vi "Update Message[ ].vi"(8 "error in (no error)":errorcluster, 10 "Message":variant, 11 "Telegram Class in":refnum<class "Telegram Class.lvclass">) -> (0 "error out":errorcluster, 3 "Telegram Class out":refnum<class "Telegram Class.lvclass">)   [LabVIEW 2015, in "Telegram Library.lvlib" / "Telegram Class.lvclass"]
doc: "Created IvanLis by LabVIEW Portal\nProfile: http://labviewportal.org/memberlist.php?mode=viewprofile&u=987\neMail: IvanLisanov@gMail.com\nTelegram: https://t.me/IvanLis"
uses:
  Telegram Class.lvclass
  JSON Library/TypeDef/Message Text.ctl
  TypeDef/Message.ctl
  Telegram Class.lvclass/Telegram Class.ctl
  Telegram Library.lvlib
  JSON Library/JSON Library.lvlib
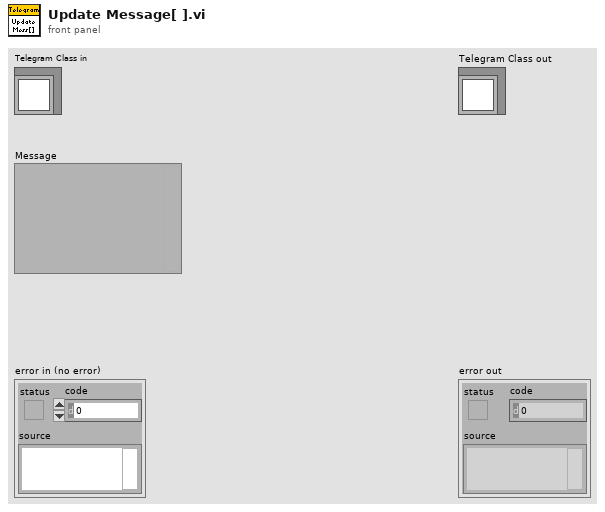
[diagram p1: front panel]
types:
  T1 = typedef "JSON Library.lvlib/Message Text.ctl" = cluster{"@type":string, "id":i64, "sender_id":cluster{"@type":string, "user_id":i64}, "chat_id":i64, "date":i64, "content":cluster{"@type":string, "text":cluster{"@type":string, "text":string}}}
  T2 = typedef "Telegram Library.lvlib/Message.ctl" = cluster{"id":i64, "chat_id":i64, "sender_user_id":i64, "date UTC":timestamp, "content_text":string}
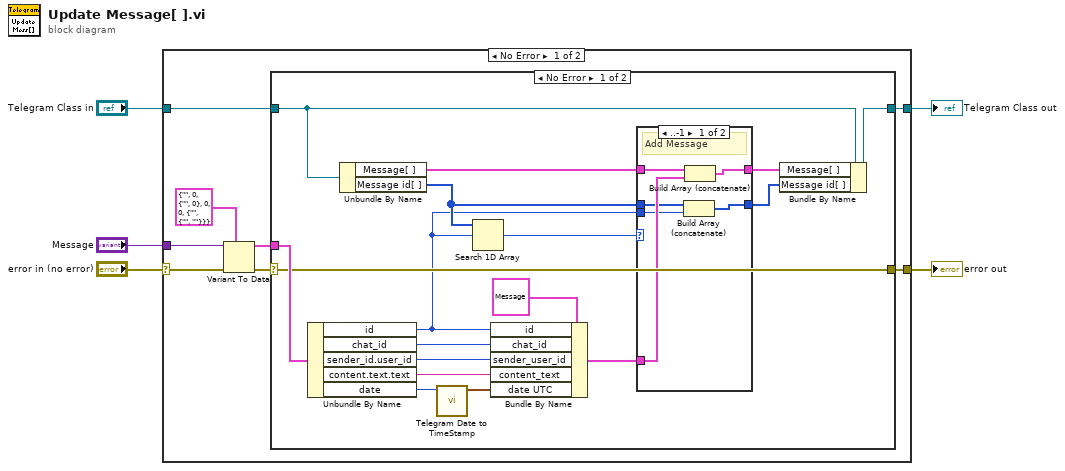
[diagram p0: block diagram]
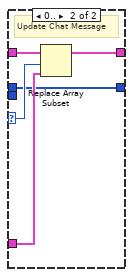
[diagram p2: hidden frame]
diagram:
  n1 = case shown="No Error" "error in (no error)" {
    selector: "error in (no error)" -> [w13 w45]
    tunnel: [w7 w45] -> w4
    tunnel: [w9 w44] -> w2
    tunnel: "Telegram Class in" -> [w10 w44]
    tunnel: "Message" -> [w11 _]
    frame No Error {
      n2 = Variant To Data(error in=w13, type=T1 {"@type"="", "id"=0, "sender_id"={"@type"="", "user_id"=0}, "chat_id"=0, "date"=0, "content"={"@type"="", "text"={"@type"="", "text"=""}}} ("Message Text"), Variant=w11) -> (data=w6:T1, error out=w8:errorcluster)
      n3 = case shown="No Error" w8 {
        selector: w8 -> [w19 w43]
        tunnel: w6 -> [w28 _]
        tunnel: [w19 w43] -> w7
        tunnel: w10 -> [w25 w42]
        tunnel: [w18 w42] -> w9
        frame No Error {
          n4 = Unbundle By Name(w28) -> ("id"=w15:i64, "chat_id"=w20:i64, "sender_id.user_id"=w29:i64, "content.text.text"=w22:string, "date"=w27:i64)
          n5 = Unbundle By Name(w25) -> ("Message[ ]"=w23:T2[], "Message id[ ]"=w16:i64[])
          n6 = call "Telegram Date to TimeStamp.vi"("date"=w27) -> ("time stamp"=w26:timestamp)  [unwired: 10 in]
          n7 = Search 1D Array(1D array=w16, element=w15) -> (index of element=w24:i32)  [unwired: 1 in]
          n8 = Bundle By Name(cluster=T2 {"id"=0, "chat_id"=0, "sender_user_id"=0, "date UTC"=timestamp(0 s since 1904-01-01), "content_text"=""} ("Message"), "id"=w15, "chat_id"=w20, "sender_user_id"=w29, "content_text"=w22, "date UTC"=w26) -> (w21:T2)
          n9 = case shown="..-1" w24 {
            selector: w24 -> [_ w39]
            tunnel: w23 -> [w36 w41]
            tunnel: w21 -> [w35 w40]
            tunnel: [w34 w38] -> w17
            tunnel: w16 -> [w33 w37]
            tunnel: w15 -> [w32 _]
            tunnel: [w31 w37] -> w14
            frame ..-1 {
              # "Add Message"
              n10 = Build Array (concatenate)(w33, w32) -> (w31:i64[])
              n11 = Build Array (concatenate)(w36, w35) -> (w34:T2[])
            }
            frame 0.. {
              # "Update Chat Message"
              n12 = Replace Array Subset(array=w41, new element=w40, index=w39) -> (w38:T2[])
            }
          }
          n13 = Bundle By Name(cluster=w25, "Message[ ]"=w17, "Message id[ ]"=w14) -> (w18:refnum<class "Telegram Class.lvclass">)
        }
        frame Error {
        }
      }
    }
    frame Error {
    }
  }
  "error out" <- w4
  "Telegram Class out" <- w2
